vi "DEMO Factory.vi"() -> ()   [LabVIEW 2011]
uses:
  Generic Plugin/Plugin Type.ctl
  Generic Plugin/Generic Plugin.lvclass
panel:
  out "Plugin color:":u32(colorbox)
  out "Plugin says:":string
  in  "Select plugin to load:":T1
  in  "stop":bool
  # "Change the ring to various values to see what each class says. See block diagram for comments."
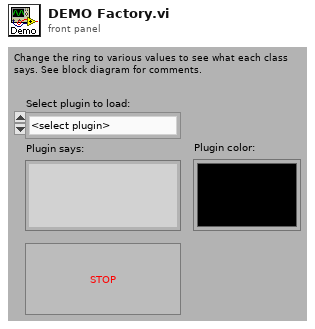
[diagram p1: front panel]
types:
  T1 = typedef "Generic Plugin.lvclass/Plugin Type.ctl" = enum16{"<select plugin>", "Orange", "Blue"}
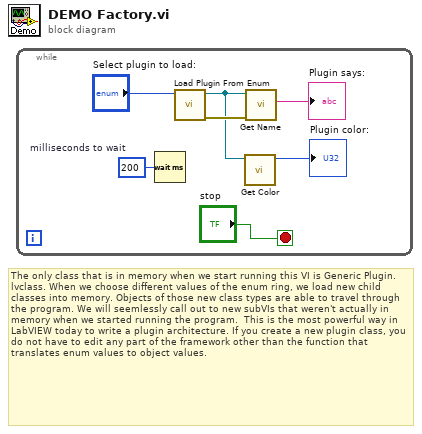
[diagram p0: block diagram]
diagram:
  # "The only class that is in memory when we start running this VI is Generic Plugin.lvclass. When we choose different values of the enum ring, we load new child classes into memory. Objects of those new class types are able to travel through the program. We will seemlessly call out to new subVIs that weren't actually in memory when we started running the program.  This is the most powerful way in LabVIEW today to write a plugin architecture. If you create a new plugin class, you do not have to edit any part of the framework other than the function that translates enum values to object values."
  n1 = while {
    stop <- "stop" stop-if-true
    w3 = u32 200  # milliseconds to wait
    n2 = Wait (ms)(milliseconds to wait=w3) -> ()  [unwired: 1 out]
    n3 = call "Load Plugin From Enum.vi"("Plugin Type"="Select plugin to load:") -> ("error out"=w5:errorcluster, "Generic Plugin.lvclass"=w2:refnum<class "Generic Plugin.lvclass">)  [unwired: 5 in]
    n4 = call-dynamic "Get Color.vi"("Generic Plugin in"=w2) -> ("Color Box"=→"Plugin color:":u32)  [unwired: 10 in]
    n5 = call-dynamic "Get Name.vi"("error in (no error)"=w5, "Generic Plugin in"=w2) -> ("Get Name"=→"Plugin says:":string)  [unwired: 7 in, 2 out]
  }
